vi "To Lower Case with Raw Name Cacher.vi"(7 "GroupName(\"\")":string, 10 "key":string) -> (1 "Raw name":string, 2 "Key in lower case":string, 6 "cacher":variant)   [LabVIEW 2017]
doc: "Converts key to lower case and caches the mapping from every lower-case name it has seen back to the original spelling, which is returned as Raw name."
uses:
  9126b41d-220b-4c2d-9ba0-52a43fc072d2.vi
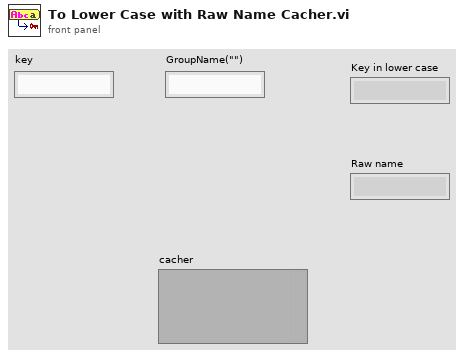
[diagram p1: front panel]
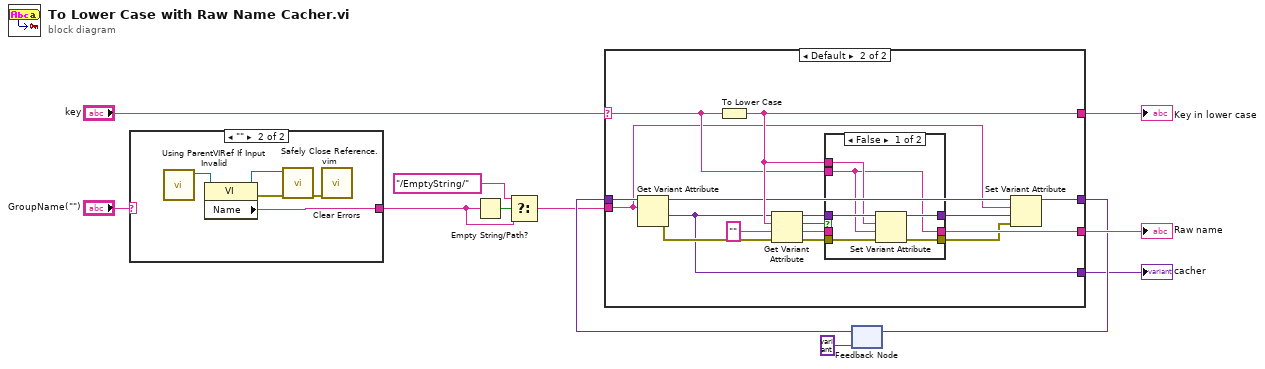
[diagram p0: block diagram]
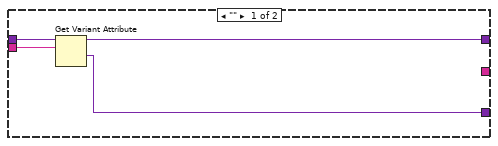
[diagram p3: hidden frame]
diagram:
  n1 = case shown="\"\"" "GroupName(\"\")" {
    selector: "GroupName(\"\")" -> [w13 _]
    tunnel: [w13 w15] -> w8
    frame "False", Default {
    }
    frame "" {
      n2 = call "Using ParentVIRef If Input Invalid.vi"() -> ("VI Ref"=w14:refnum<vi>)  [unwired: 6 in, 1 out]
      n3 = property class="VI"(reference=w14) -> (reference out=w17:refnum<vi>, error out=w16:errorcluster, "Name"=w15:string)  [unwired: 1 in]
      n4 = call "Safely Close Reference.vim"("error in (no error)"=w16, "Reference"=w17) -> ("error out"=w18:errorcluster)  [unwired: 9 in]
      n5 = call <vilib>:"Clear Errors.vi"("error in (no error)"=w18) -> ()  [unwired: 5 in, 2 out]
    }
  }
  n6 = Empty String/Path?(string/path=w8) -> (empty?=w7:bool)
  n7 = Select(t="/EmptyString/", s=w7, f=w8) -> (s? t:f=w4:string)
  n8 = feedback #1(variant) -> (w5:variant)
  n9 = case shown="Default" "key" {
    selector: "key" -> [_ w37]
    tunnel: [_ w38] -> w12
    tunnel: [_ w36] -> w10
    tunnel: w5 -> [w21 w30]
    tunnel: w4 -> [w22 w27]
    tunnel: [w20 w24] -> w3
    tunnel: [w19 w23] -> w2
    frame "" {
      n10 = Get Variant Attribute(Variant=w21, name=w22) -> (duplicate Variant=w20:variant, value=w19:variant)  [unwired: 2 in, 2 out]
    }
    frame Default {
      n11 = Get Variant Attribute(Variant=w30, name=w27) -> (duplicate Variant=w29:variant, value=w23:variant, error out=w26:errorcluster)  [unwired: 2 in, 1 out]
      n12 = To Lower Case(string=w37) -> (all lower case string=w38:string)
      n13 = Get Variant Attribute(Variant=w23, name=w38, default value (empty Variant)="", error in=w26) -> (duplicate Variant=w35:variant, found=w33:bool, value=w32:string, error out=w31:errorcluster)
      n14 = case shown="False" w33 {
        tunnel: w35 -> [w44 w47]
        tunnel: w38 -> [w43 _]
        tunnel: w37 -> [w40 _]
        tunnel: w32 -> [_ w46]
        tunnel: w31 -> [w42 w45]
        tunnel: [w41 w47] -> w28
        tunnel: [w40 w46] -> w36
        tunnel: [w39 w45] -> w25
        frame False {
          n15 = Set Variant Attribute(Variant=w44, name=w43, value=w40, error in=w42) -> (Variant out=w41:variant, error out=w39:errorcluster)  [unwired: 1 out]
        }
        frame True {
        }
      }
      n16 = Set Variant Attribute(Variant=w29, name=w27, value=w28, error in=w25) -> (Variant out=w24:variant)  [unwired: 2 out]
    }
  }
  "Key in lower case" <- w12
  "Raw name" <- w10
  "cacher" <- w2
  n17 = feedback-in #1(w3) -> ()
